vi "convert to unicode.vi"(11 "System String":string) -> (3 "UTF8 String":string)   [LabVIEW 2013, in "lvnano.lvlib"]
uses:
  lvnano.lvlib
  lvnanomsg.dll
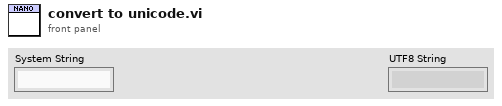
[diagram p1: front panel]
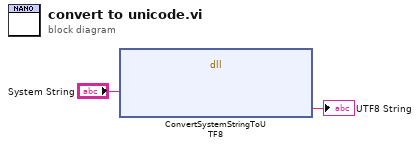
[diagram p0: block diagram]
diagram:
  n1 = dll-call lib="C:/Users/Daniel/Documents/nanomsg/lvnano/lvnanomsg.*" fn="ConvertSystemStringToUTF8"("System String"="System String") -> ("UTF8 String"=→"UTF8 String":string)  [unwired: 6 in, 2 out]
